vi "is_int.vi"(11 "data in":string) -> (1 "confirmed?":bool, 3 "data out":variant)   [LabVIEW 2020, in "configuration-data.lvclass"]
uses:
  configuration-data.lvclass
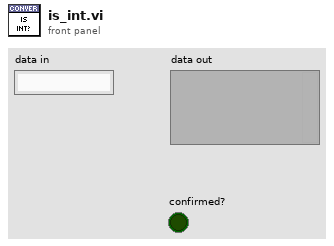
[diagram p1: front panel]
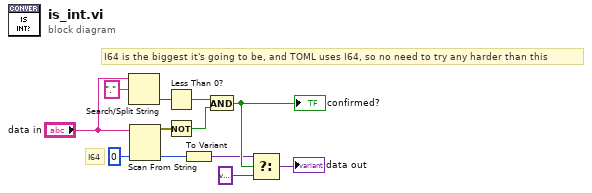
[diagram p0: block diagram]
diagram:
  # "I64"
  # "I64 is the biggest it's going to be, and TOML uses I64, so no need to try any harder than this"
  n1 = Search/Split String(string="data in", search string/char (-)=".") -> (offset of match=w8:i32)  [unwired: 1 in, 2 out]
  n2 = Scan From String(input string="data in", default 1=i64 0 ("default value 1")) -> (error out=w11:errorcluster, output 1=w4:i64)  [unwired: 3 in, 2 out]
  n3 = Less Than 0?(x=w8) -> (x < 0?=w7:bool)
  n4 = Not(x=w11) -> (.not. x?=w6:bool)
  n5 = To Variant(anything=w4) -> (Variant=w2:variant)
  n6 = And(x=w7, y=w6) -> (x .and. y?=w5:bool)
  "confirmed?" <- w5
  n7 = Select(t=w2, s=w5, f=variant) -> (s? t:f=→"data out":variant)
